vi "Create_Object.vi"(8 "error in (no error)":errorcluster, 9 "Terminal Map in":map{string, T1}(c390), 10 "owner refnum":variant, 11 "Structure in":refnum<class "Structure.lvclass">) -> (0 "error out":errorcluster, 1 "Terminal Map Out":map{string, T1}(c390), 3 "Structure out":refnum<class "Structure.lvclass">)   [LabVIEW 2025, in "Structure.lvclass"]
uses:
  Structure.lvclass
  Controls/Terminal.ctl
  Node.lvclass/Node.ctl
  Node.lvclass
  Structure.lvclass/Structure.ctl
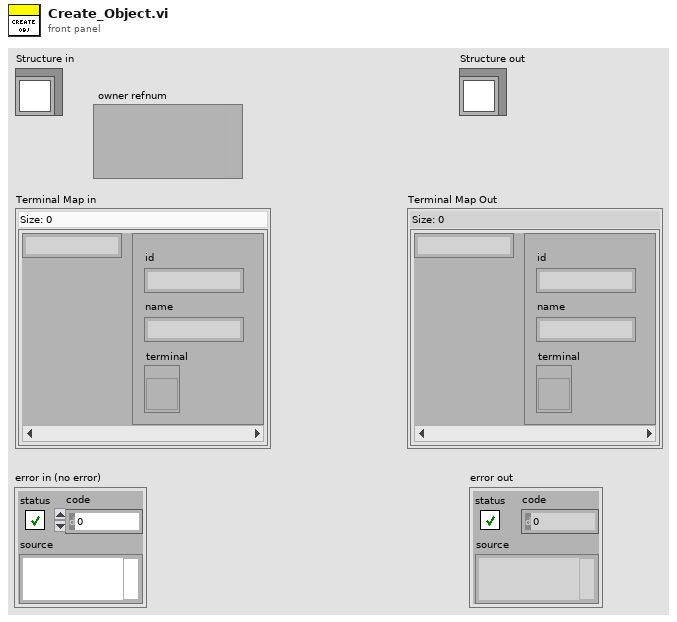
[diagram p1: front panel]
types:
  T1 = typedef "Terminal.ctl" = cluster{"id":string, "name":string, "terminal":refnum<vi>}
  T2 = typedef "Subdiagram.ctl" = cluster{"diagram":refnum<vi>, "selector":string, "uuid":string}
  T3 = typedef "LVPointTypeDef.ctl" = cluster{"Horizontal":i16, "Vertical":i16}
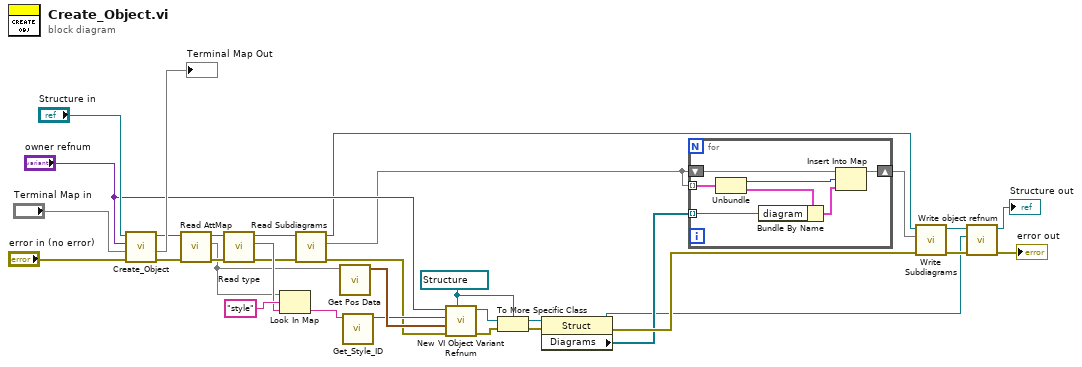
[diagram p0: block diagram]
diagram:
  w17 = refnum<vi> refnum ("vi object class")
  n1 = call-parent "Create_Object.vi"("error in (no error)"="error in (no error)", "Terminal Map in"="Terminal Map in", "owner refnum"="owner refnum", "Node in"="Structure in") -> ("error out"=w27:errorcluster, "Terminal Map Out"=→"Terminal Map Out":map{string, T1}, "Node out"=w26:refnum<class "Structure.lvclass">)  [unwired: 5 in]
  n2 = call "Read AttMap.vi"("error in (no error)"=w27, "Node in"=w26) -> ("error out"=w28:errorcluster, "AttMap"=w23:map{string, string}, "Node out"=w29:refnum<class "Structure.lvclass">)  [unwired: 7 in]
  n3 = call "Read type.vi"("error in (no error)"=w28, "Node in"=w29) -> ("error out"=w14:errorcluster, "type"=w24:string, "Node out"=w13:refnum<class "Structure.lvclass">)  [unwired: 7 in]
  n4 = Look In Map(map=w23, key="style", default value=w24) -> (value=w22:string)  [unwired: 1 out]
  n5 = call-dynamic "Read Subdiagrams.vi"("error in (no error)"=w14, "Structure in"=w13) -> ("error out"=w12:errorcluster, "Subdiagrams"=w1:map{u64, T2}, "Structure out"=w2:refnum<class "Structure.lvclass">)  [unwired: 7 in]
  n6 = call "Get Pos Data.vi"("AttMap"=w23) -> ("Position"=w21:T3)  [unwired: 10 in]
  n7 = call "Get_Style_ID.vi"("Style"=w22) -> ("style"=w20:i32)  [unwired: 8 in, 2 out]
  n8 = call "New VI Object Variant Refnum.vi"("vi object class"=w17, "error in (no error)"=w12, "location"=w21, "style"=w20, "owner refnum"="owner refnum") -> ("error out"=w16:errorcluster, "object refnum"=w18:refnum<vi>)  [unwired: 5 in]
  n9 = To More Specific Class(target class=w17, reference=w18, error in=w16) -> (specific class reference=w15:refnum<vi>, error out=w10:errorcluster)
  n10 = property class="Struct"(reference=w15, error in=w10) -> (reference out=w3:refnum<vi>, error out=w9:errorcluster, "Diagrams"=w8:refnum<vi>[])
  n11 = for {
    tunnel: w8 -> [w34] mode=indexing
    tunnel: w1 -> [w40] mode=indexing
    shift-right: [w35] -> w11
    shift-left: w1 -> [w38]
    n12 = Unbundle(w40) -> ("Numeric"=w36:u64, "Subdiagram"=w39:T2)
    n13 = Bundle By Name(cluster=w39, "diagram"=w34) -> (w37:T2)
    n14 = Insert Into Map(map in=w38, key=w36, value=w37) -> (map out=w35:map{u64, T2})  [unwired: 2 out]
  }
  n15 = call-dynamic "Write Subdiagrams.vi"("error in (no error)"=w9, "Subdiagrams"=w11, "Structure in"=w2) -> ("error out"=w7:errorcluster, "Structure out"=w6:refnum<class "Structure.lvclass">)  [unwired: 7 in]
  n16 = call-dynamic "Write object refnum.vi"("error in (no error)"=w7, "object refnum"=w3, "Node in"=w6) -> ("error out"=→"error out":errorcluster, "Node out"=→"Structure out":refnum<class "Structure.lvclass">)  [unwired: 7 in]
